vi "AddCartesianVectors.vi"(8 "error in (no error)":errorcluster, 10 "CartesianVector in B":refnum<class "CartesianVector.lvclass">, 11 "CartesianVector in A":refnum<class "CartesianVector.lvclass">) -> (0 "error out":errorcluster, 1 "Y (North)":dbl, 2 "X (East)":dbl, 3 "CartesianVector out":refnum<class "CartesianVector.lvclass">)   [LabVIEW 2013, in "CartesianVector.lvclass"]
uses:
  CartesianVector.lvclass
  CartesianVector.lvclass/CartesianVector.ctl
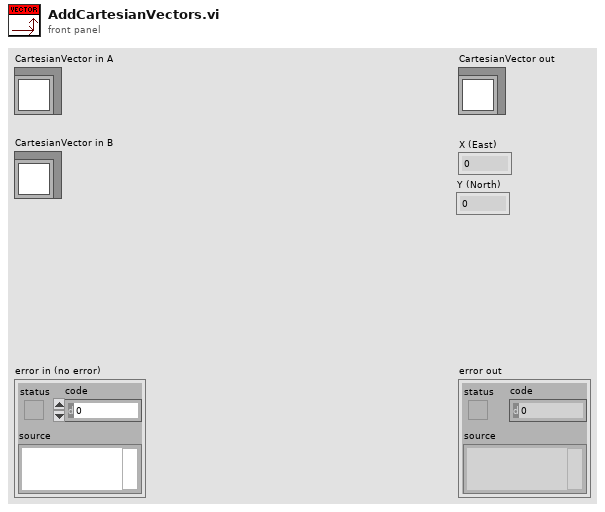
[diagram p1: front panel]
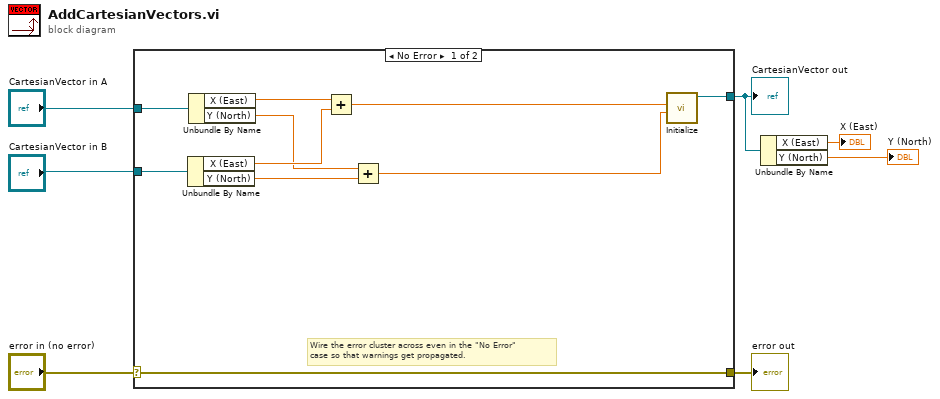
[diagram p0: block diagram]
diagram:
  n1 = case shown="No Error" "error in (no error)" {
    selector: "error in (no error)" -> [w17 w19]
    tunnel: [w17 w19] -> w6
    tunnel: [w16 w18] -> w3
    tunnel: "CartesianVector in A" -> [w15 w18]
    tunnel: "CartesianVector in B" -> [w14 _]
    frame No Error {
      # "Wire the error cluster across even in the \"No Error\"\ncase so that warnings get propagated."
      n2 = Unbundle By Name(w14) -> ("X (East)"=w12:dbl, "Y (North)"=w11:dbl)
      n3 = Unbundle By Name(w15) -> ("X (East)"=w13:dbl, "Y (North)"=w10:dbl)
      n4 = Add(x=w13, y=w12) -> (x+y=w8:dbl)
      n5 = Add(x=w10, y=w11) -> (x+y=w9:dbl)
      n6 = call "Initialize.vi"("Y (North)"=w9, "X (East)"=w8) -> ("CartesianVector out"=w16:refnum<class "CartesianVector.lvclass">)  [unwired: 8 in, 1 out]
    }
    frame Error {
    }
  }
  "error out" <- w6
  "CartesianVector out" <- w3
  n7 = Unbundle By Name(w3) -> ("X (East)"=→"X (East)":dbl, "Y (North)"=→"Y (North)":dbl)
